vi "USB2CANFD_Test.vi"() -> ()   [LabVIEW 2010]
panel:
  out "Get Msg Num":i32
  out "pCanGetMsg OUT":T1(array[cluster])
  in  "stop":bool
  out "Success Sended Msg Num":i32
  in  "pCanSendMsg":T2={"ID"=1, "DLC"=8, "Flags"=0, "__Res0"=0, "__Res1"=0, "TimeStamp"=0, "Data[0]"=1, "Data[1]"=2, "Data[2]"=3, "Data[3]"=4, "Data[4]"=5, "Data[5]"=6, "Data[6]"=7, "Data[7]"=8, "Data[8]"=0, "Data[9]"=0, "Data[10]"=0, "Data[11]"=0, "Data[12]"=0, "Data[13]"=0, "Data[14]"=0, "Data[15]"=0, "Data[16]"=0, "Data[17]"=0, "Data[18]"=0, "Data[19]"=0, "Data[20]"=0, "Data[21]"=0, "Data[22]"=0, "Data[23]"=0, "Data[24]"=0, "Data[25]"=0, "Data[26]"=0, "Data[27]"=0, "Data[28]"=0, "Data[29]"=0, "Data[30]"=0, "Data[31]"=0, "Data[32]"=0, "Data[33]"=0, "Data[34]"=0, "Data[35]"=0, "Data[36]"=0, "Data[37]"=0, "Data[38]"=0, "Data[39]"=0, "Data[40]"=0, "Data[41]"=0, "Data[42]"=0, "Data[43]"=0, "Data[44]"=0, "Data[45]"=0, "Data[46]"=0, "Data[47]"=0, "Data[48]"=0, "Data[49]"=0, "Data[50]"=0, "Data[51]"=0, "Data[52]"=0, "Data[53]"=0, "Data[54]"=0, "Data[55]"=0, "Data[56]"=0, "Data[57]"=0, "Data[58]"=0, "Data[59]"=0, "Data[60]"=0, "Data[61]"=0, "Data[62]"=0, "Data[63]"=0} {"ID" format="%x"; "Data[1]" format="%x"; "Data[2]" format="%x"}
  in  "CAN Channel":u8(ring) items=["CAN1", "CAN2"]
  in  "Device Index":i32(ring) items=["0", "1", "2", "3", "4", "5"]
  in  "pCanGetMsg":T2
  in  "pCanConfig":T3={"Mode"=1, "ISOCRCEnable"=0, "RetrySend"=1, "ResEnable"=1, "NBT_BRP"=1, "NBT_SEG1"=63, "NBT_SEG2"=16, "NBT_SJW"=16, "DBT_BRP"=1, "DBT_SEG1"=15, "DBT_SEG2"=4, "DBT_SJW"=4, "__Res0[0]"=0, "__Res0[1]"=0, "__Res0[2]"=0, "__Res0[3]"=0, "__Res0[4]"=0, "__Res0[5]"=0, "__Res0[6]"=0, "__Res0[7]"=0}
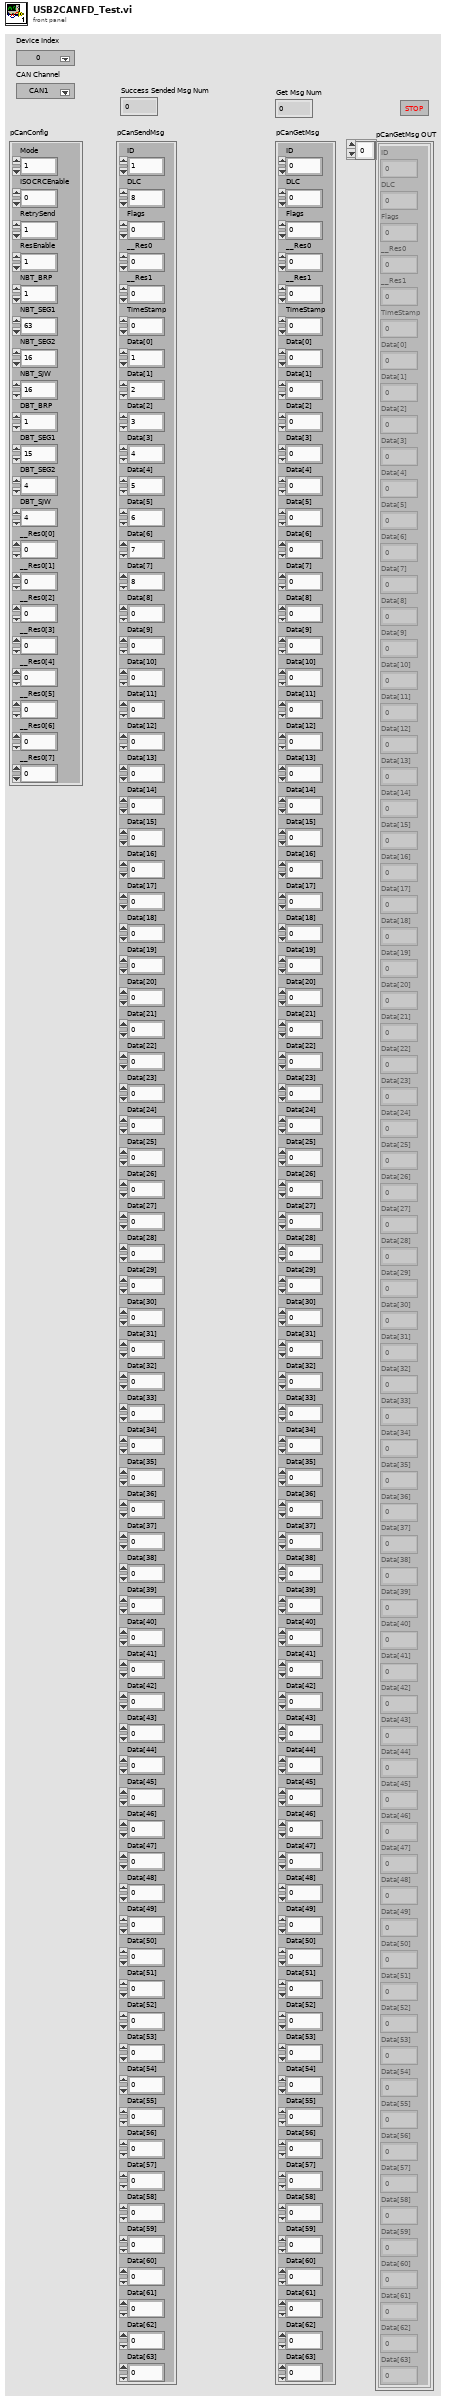
[diagram p1: front panel]
types:
  T1 = cluster{"ID":u32, "DLC":u8, "Flags":u8, "__Res0":u8, "__Res1":u8, "TimeStamp":u32, "Data[0]":u8, "Data[1]":u8, "Data[2]":u8, "Data[3]":u8, "Data[4]":u8, "Data[5]":u8, "Data[6]":u8, "Data[7]":u8, "Data[8]":u8, "Data[9]":u8, "Data[10]":u8, "Data[11]":u8, "Data[12]":u8, "Data[13]":u8, "Data[14]":u8, "Data[15]":u8, "Data[16]":u8, "Data[17]":u8, "Data[18]":u8, "Data[19]":u8, "Data[20]":u8, "Data[21]":u8, "Data[22]":u8, "Data[23]":u8, "Data[24]":u8, "Data[25]":u8, "Data[26]":u8, "Data[27]":u8, "Data[28]":u8, "Data[29]":u8, "Data[30]":u8, "Data[31]":u8, "Data[32]":u8, "Data[33]":u8, "Data[34]":u8, "Data[35]":u8, "Data[36]":u8, "Data[37]":u8, "Data[38]":u8, "Data[39]":u8, "Data[40]":u8, "Data[41]":u8, "Data[42]":u8, "Data[43]":u8, "Data[44]":u8, "Data[45]":u8, "Data[46]":u8, "Data[47]":u8, "Data[48]":u8, "Data[49]":u8, "Data[50]":u8, "Data[51]":u8, "Data[52]":u8, "Data[53]":u8, "Data[54]":u8, "Data[55]":u8, "Data[56]":u8, "Data[57]":u8, "Data[58]":u8, "Data[59]":u8, "Data[60]":u8, "Data[61]":u8, "Data[62]":u8, "Data[63]":u8}[]
  T2 = cluster{"ID":u32, "DLC":u8, "Flags":u8, "__Res0":u8, "__Res1":u8, "TimeStamp":u32, "Data[0]":u8, "Data[1]":u8, "Data[2]":u8, "Data[3]":u8, "Data[4]":u8, "Data[5]":u8, "Data[6]":u8, "Data[7]":u8, "Data[8]":u8, "Data[9]":u8, "Data[10]":u8, "Data[11]":u8, "Data[12]":u8, "Data[13]":u8, "Data[14]":u8, "Data[15]":u8, "Data[16]":u8, "Data[17]":u8, "Data[18]":u8, "Data[19]":u8, "Data[20]":u8, "Data[21]":u8, "Data[22]":u8, "Data[23]":u8, "Data[24]":u8, "Data[25]":u8, "Data[26]":u8, "Data[27]":u8, "Data[28]":u8, "Data[29]":u8, "Data[30]":u8, "Data[31]":u8, "Data[32]":u8, "Data[33]":u8, "Data[34]":u8, "Data[35]":u8, "Data[36]":u8, "Data[37]":u8, "Data[38]":u8, "Data[39]":u8, "Data[40]":u8, "Data[41]":u8, "Data[42]":u8, "Data[43]":u8, "Data[44]":u8, "Data[45]":u8, "Data[46]":u8, "Data[47]":u8, "Data[48]":u8, "Data[49]":u8, "Data[50]":u8, "Data[51]":u8, "Data[52]":u8, "Data[53]":u8, "Data[54]":u8, "Data[55]":u8, "Data[56]":u8, "Data[57]":u8, "Data[58]":u8, "Data[59]":u8, "Data[60]":u8, "Data[61]":u8, "Data[62]":u8, "Data[63]":u8}
  T3 = cluster{"Mode":u8, "ISOCRCEnable":u8, "RetrySend":u8, "ResEnable":u8, "NBT_BRP":u8, "NBT_SEG1":u8, "NBT_SEG2":u8, "NBT_SJW":u8, "DBT_BRP":u8, "DBT_SEG1":u8, "DBT_SEG2":u8, "DBT_SJW":u8, "__Res0[0]":u8, "__Res0[1]":u8, "__Res0[2]":u8, "__Res0[3]":u8, "__Res0[4]":u8, "__Res0[5]":u8, "__Res0[6]":u8, "__Res0[7]":u8}
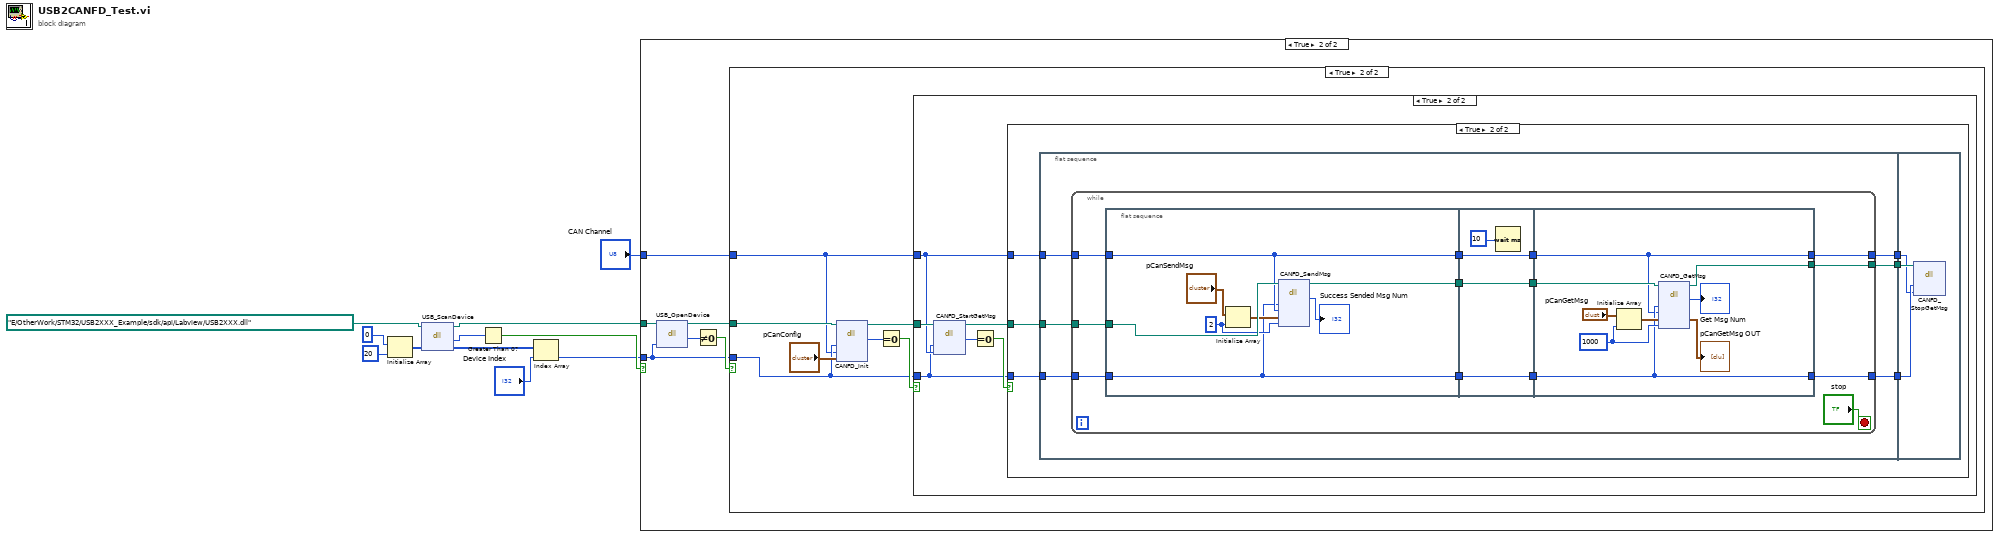
[diagram p0: block diagram]
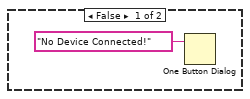
[diagram p2: hidden frame]
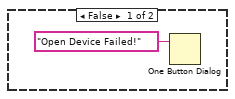
[diagram p3: hidden frame]
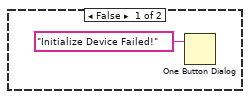
[diagram p4: hidden frame]
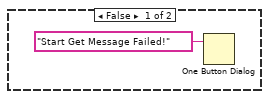
[diagram p5: hidden frame]
diagram:
  n1 = Initialize Array(0, 20 ("dimension size")) -> (w11:i32[])
  n2 = dll-call lib="E:/OtherWork/STM32/USB2XXX_Example/sdk/api/Labview/USB2XXX.dll" fn="USB_ScanDevice"(path in=path "E:/OtherWork/STM32/USB2XXX_Example/sdk/api/Labview/USB2XXX.dll", "pDevNum"=w11) -> (path out=w1:path, "return type"=w7:i32, "pDevNum"=w8:i32[])  [unwired: 2 in, 1 out]
  n3 = Greater Than 0?(x=w7) -> (x > 0?=w6:bool)
  n4 = Index Array(array=w8, index="Device Index") -> (element=w4:i32)
  n5 = case shown="True" w6 {
    tunnel: w4 -> [_ w15]
    tunnel: w1 -> [_ w16]
    tunnel: "CAN Channel" -> [_ w14]
    frame False {
      n6 = One Button Dialog(message="No Device Connected!") -> ()  [unwired: 1 in, 1 out]
    }
    frame True {
      n7 = dll-call lib="E:/OtherWork/STM32/USB2XXX_Example/sdk/api/Labview/USB2XXX.*" fn="USB_OpenDevice"(path in=w16, "DevHandle"=w15) -> (path out=w13:path, "return type"=w18:u8)  [unwired: 3 in, 1 out]
      n8 = Not Equal To 0?(x=w18) -> (x != 0?=w17:bool)
      n9 = case shown="True" w17 {
        tunnel: w13 -> [_ w26]
        tunnel: w15 -> [_ w21]
        tunnel: w14 -> [_ w20]
        frame False {
          n10 = One Button Dialog(message="Open Device Failed!") -> ()  [unwired: 1 in, 1 out]
        }
        frame True {
          n11 = dll-call lib="E:/OtherWork/STM32/USB2XXX_Example/sdk/api/Labview/USB2XXX.*" fn="CANFD_Init"(path in=w26, "DevHandle"=w21, "CANIndex"=w20, "pCanConfig"="pCanConfig") -> (path out=w22:path, "return type"=w24:i32)  [unwired: 5 in, 1 out]
          n12 = Equal To 0?(x=w24) -> (x = 0?=w23:bool)
          n13 = case shown="True" w23 {
            tunnel: w22 -> [_ w33]
            tunnel: w21 -> [_ w28]
            tunnel: w20 -> [_ w29]
            frame False {
              n14 = One Button Dialog(message="Initialize Device Failed!") -> ()  [unwired: 1 in, 1 out]
            }
            frame True {
              n15 = dll-call lib="E:/OtherWork/STM32/USB2XXX_Example/sdk/api/Labview/USB2XXX.*" fn="CANFD_StartGetMsg"(path in=w33, "DevHandle"=w28, "CANIndex"=w29) -> (path out=w30:path, "return type"=w32:i32)  [unwired: 4 in, 1 out]
              n16 = Equal To 0?(x=w32) -> (x = 0?=w31:bool)
              n17 = case shown="True" w31 {
                tunnel: w30 -> [_ w40]
                tunnel: w29 -> [_ w39]
                tunnel: w28 -> [_ w38]
                frame False {
                  n18 = One Button Dialog(message="Start Get Message Failed!") -> ()  [unwired: 1 in, 1 out]
                }
                frame True {
                  n19 = flat-sequence {
                    tunnel: w40 -> [w46]
                    tunnel: w39 -> [w45]
                    tunnel: w38 -> [w44]
                    tunnel: [w43] -> w37
                    tunnel: [w42] -> w36
                    tunnel: [w41] -> w35
                    tunnel: w37 -> [w83]
                    tunnel: w36 -> [w82]
                    tunnel: w35 -> [w81]
                    frame #0 {
                      n20 = while {
                        tunnel: w46 -> [w59]
                        tunnel: w45 -> [w58]
                        tunnel: w44 -> [w57]
                        tunnel: [w49] -> w43
                        tunnel: [w48] -> w42
                        tunnel: [w47] -> w41
                        stop <- "stop" stop-if-true
                        n21 = flat-sequence {
                          tunnel: w59 -> [w67]
                          tunnel: w58 -> [w62]
                          tunnel: w57 -> [w61]
                          tunnel: [w62] -> w55
                          tunnel: [w61] -> w53
                          tunnel: [w60] -> w51
                          tunnel: w55 -> [w70]
                          tunnel: [w70] -> w54
                          tunnel: w53 -> [w69]
                          tunnel: [w69] -> w52
                          tunnel: w51 -> [w68]
                          tunnel: [w68] -> w50
                          tunnel: w54 -> [w72]
                          tunnel: w52 -> [w73]
                          tunnel: w50 -> [w77]
                          tunnel: [w74] -> w49
                          tunnel: [w73] -> w48
                          tunnel: [w72] -> w47
                          frame #0 {
                            w64 = u32 2 ("dimension size")
                            n22 = Initialize Array("pCanSendMsg", w64) -> (w65:T1)
                            n23 = dll-call lib="E:/OtherWork/STM32/USB2XXX_Example/sdk/api/Labview/USB2XXX.*" fn="CANFD_SendMsg"(path in=w67, "DevHandle"=w61, "CANIndex"=w62, "pCanSendMsg"=w65, "SendMsgNum"=w64) -> (path out=w60:path, "return type"=→"Success Sended Msg Num":i32)  [unwired: 6 in, 1 out]
                          }
                          frame #1 {
                            n24 = Wait (ms)(milliseconds to wait=u32 10 ("等待时间（毫秒）")) -> ()  [unwired: 1 out]
                          }
                          frame #2 {
                            w78 = 1000 ("BufferSize")
                            n25 = Initialize Array("pCanGetMsg", w78) -> (w79:T1)
                            n26 = dll-call lib="E:/OtherWork/STM32/USB2XXX_Example/sdk/api/Labview/USB2XXX.dll" fn="CANFD_GetMsg"(path in=w77, "DevHandle"=w73, "CANIndex"=w72, "pCanGetMsg"=w79, "BufferSize"=w78) -> (path out=w74:path, "return type"=→"Get Msg Num":i32, "pCanGetMsg"=→"pCanGetMsg OUT":T1)  [unwired: 5 in, 1 out]
                          }
                        }
                      }
                    }
                    frame #1 {
                      n27 = dll-call lib="E:/OtherWork/STM32/USB2XXX_Example/sdk/api/Labview/USB2XXX.*" fn="CANFD_StopGetMsg"(path in=w83, "DevHandle"=w82, "CANIndex"=w81) -> ()  [unwired: 5 in, 2 out]
                    }
                  }
                }
              }
            }
          }
        }
      }
    }
  }
